vi "AlliGator [Z] to Z Plot.vi"(8 "Error In":errorcluster, 9 "Phasor Graph Slide (-1: last)":i32=-1, 10 "Single Point Display? (F)":bool, 11 "[Calibrated Phasor]":T1[](array[typedef])) -> (0 "Error Out":errorcluster, 3 "Calibrated Phasor Plot":cluster{"Array":dbl[], "Array":dbl[]})   [LabVIEW 2021, in "AlliGator Phasor Calibration.lvlib"]
doc: "Returns full plot of the series of phasors, or only one if <B>Single Point Display</B> = True.\n\nThe <B>Phasor Graph Slide</B> sepecifies which point to display."
uses:
  AlliGator Phasor Calibration.lvlib
  Phasor/Phasor (g, s).ctl
  ac0ce6f8-85b7-41c8-85c3-d4d04f84f1e4.vi
  18744cc5-2d74-4d38-ba8f-23fcda318c75.vi
  Arrays/Signed Array Index.vi
  Phasor/Phasor.lvlib
panel:
  # "see the AlliGator License on the block diagram (Ctrl+E or Window:Show Block Diagram)"
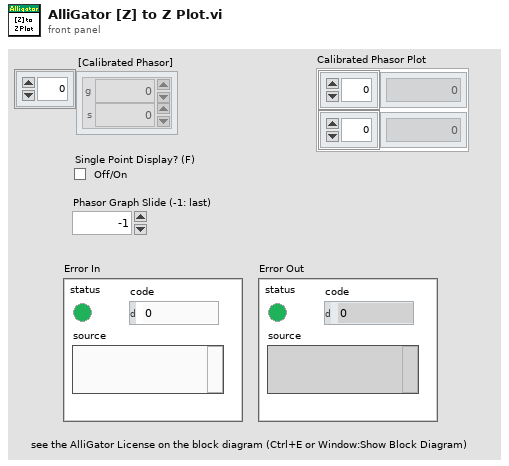
[diagram p1: front panel]
types:
  T1 = typedef "Phasor.lvlib/Phasor (g, s).ctl" = cluster{"g":dbl, "s":dbl}
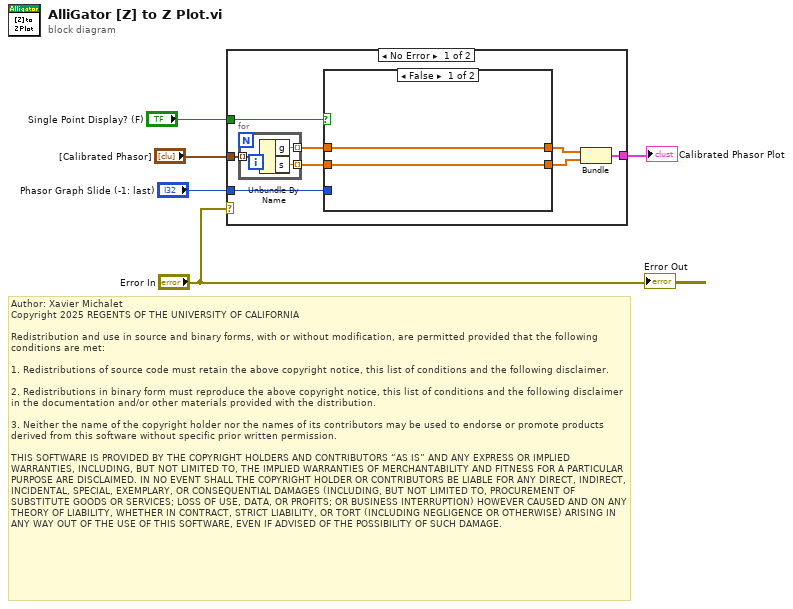
[diagram p0: block diagram]
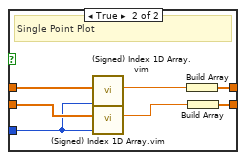
[diagram p2: hidden frame]
diagram:
  # "Author: Xavier Michalet\nCopyright 2025 REGENTS OF THE UNIVERSITY OF CALIFORNIA\n\nRedistribution and use in source and binary forms, with or without modification, are permitted provided that the following conditions are met:\n\n1. Redistributions of source code must retain the above copyright notice, this list of conditions and the following disclaimer.\n\n2. Redistributions in binary form must reproduce the above copyright notice, this list of conditions and the following disclaimer in the documentation and/or other materials provided with the distribution.\n\n3. Neither the name of the copyright holder nor the names of its contributors may be used to endorse or promote products derived from this software without specific prior written permission.\n\nTHIS SOFTWARE IS PROVIDED BY THE COPYRIGHT HOLDERS AND CONTRIBUTORS “AS IS” AND ANY EXPRESS OR IMPLIED WARRANTIES, INCLUDING, BUT NOT LIMITED TO, THE IMPLIED WARRANTIES OF MERCHANTABILITY AND FITNESS FOR A PARTICULAR PURPOSE ARE DISCLAIMED. IN NO EVENT SHALL THE COPYRIGHT HOLDER OR CONTRIBUTORS BE LIABLE FOR ANY DIRECT, INDIRECT, INCIDENTAL, SPECIAL, EXEMPLARY, OR CONSEQUENTIAL DAMAGES (INCLUDING, BUT NOT LIMITED TO, PROCUREMENT OF SUBSTITUTE GOODS OR SERVICES; LOSS OF USE, DATA, OR PROFITS; OR BUSINESS INTERRUPTION) HOWEVER CAUSED AND ON ANY THEORY OF LIABILITY, WHETHER IN CONTRACT, STRICT LIABILITY, OR TORT (INCLUDING NEGLIGENCE OR OTHERWISE) ARISING IN ANY WAY OUT OF THE USE OF THIS SOFTWARE, EVEN IF ADVISED OF THE POSSIBILITY OF SUCH DAMAGE."
  n1 = case shown="No Error" "Error In" {
    tunnel: [w13 _] -> w5
    tunnel: "Phasor Graph Slide (-1: last)" -> [w10 _]
    tunnel: "Single Point Display? (F)" -> [w9 _]
    tunnel: "[Calibrated Phasor]" -> [w8 _]
    frame No Error {
      n2 = for {
        tunnel: w8 -> [w25] mode=indexing
        tunnel: [w24] -> w7 mode=indexing
        tunnel: [w23] -> w6 mode=indexing
        n3 = Unbundle By Name(w25) -> ("g"=w24:dbl, "s"=w23:dbl)
      }
      n4 = case shown="False" w9 {
        tunnel: w10 -> [_ w20]
        tunnel: [w15 w17] -> w11
        tunnel: [w14 w16] -> w12
        tunnel: w7 -> [w15 w22]
        tunnel: w6 -> [w14 w21]
        frame False {
        }
        frame True {
          # "Single Point Plot"
          n5 = call "(Signed) Index 1D Array.vim"("Signed Index"=w20, "Array"=w22) -> ("Array Element"=w19:dbl)  [unwired: 9 in]
          n6 = call "(Signed) Index 1D Array.vim"("Signed Index"=w20, "Array"=w21) -> ("Array Element"=w18:dbl)  [unwired: 9 in]
          n7 = Build Array(w19) -> (w17:dbl[])
          n8 = Build Array(w18) -> (w16:dbl[])
        }
      }
      n9 = Bundle(w11, w12) -> (w13:cluster{dbl[], dbl[]})  [unwired: 1 in]
    }
    frame Error {
    }
  }
  "Calibrated Phasor Plot" <- w5
  "Error Out" <- "Error In"
